vi "test_Packet_SimplePipelineResult.vi"(8 "error in (no error)":errorcluster) -> (0 "error out":errorcluster, 3 "Test Passed":bool)   [LabVIEW 2019]
uses:
  PhotonVisionLib/TypeDef/PhotonTrackedTargetType.ctl
  PhotonVisionLib/TypeDef/TargetCornerType.ctl
  <vilib>/Rock Robotics/WPI/ThirdParty/JAS_Junk/TrajLib/TRANSFORM2D.ctl
  <vilib>/Rock Robotics/WPI/ThirdParty/JAS_Junk/TrajLib/TRANSLATION2D.ctl
  <vilib>/Rock Robotics/WPI/ThirdParty/JAS_Junk/TrajLib/ROTATION2D.ctl
  PhotonVisionLib/PhotonVisionLib.lvlib
  <vilib>/Rock Robotics/WPI/ThirdParty/JAS_Junk/TrajLib/Trajectory_Library.lvlib
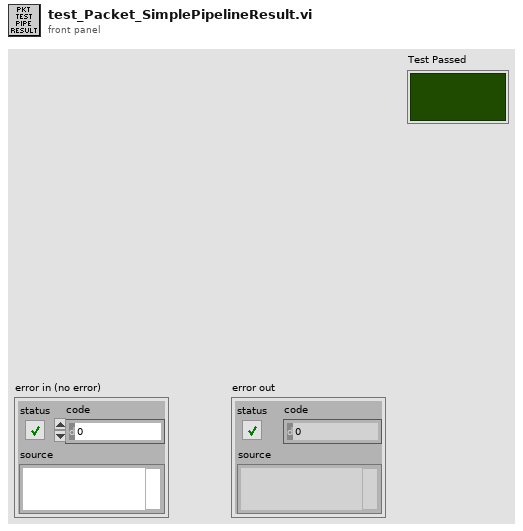
[diagram p1: front panel]
types:
  T1 = typedef "PhotonVisionLib.lvlib/PhotonTrackedTargetType.ctl" = cluster{"Yaw":dbl, "Pitch":dbl, "Area":dbl, "Skew":dbl, "TargetCorners":T2[], "CameraToTarget":T3}
  T2 = typedef "PhotonVisionLib.lvlib/TargetCornerType.ctl" = cluster{"X":dbl, "Y":dbl}
  T3 = typedef "Trajectory_Library.lvlib/TRANSFORM2D.ctl" = cluster{"TRANSLATION":T4, "ROTATION":T5}
  T4 = typedef "Trajectory_Library.lvlib/TRANSLATION2D.ctl" = cluster{"X":dbl, "Y":dbl}
  T5 = typedef "Trajectory_Library.lvlib/ROTATION2D.ctl" = cluster{"VALUE":dbl, "COS":dbl, "SIN":dbl}
  T6 = typedef "PhotonVisionLib.lvlib/PhotonPipelineResultType.ctl" = cluster{"TargetCount":i32, "Latency_MilliSec":dbl, "Targets":T1[]}
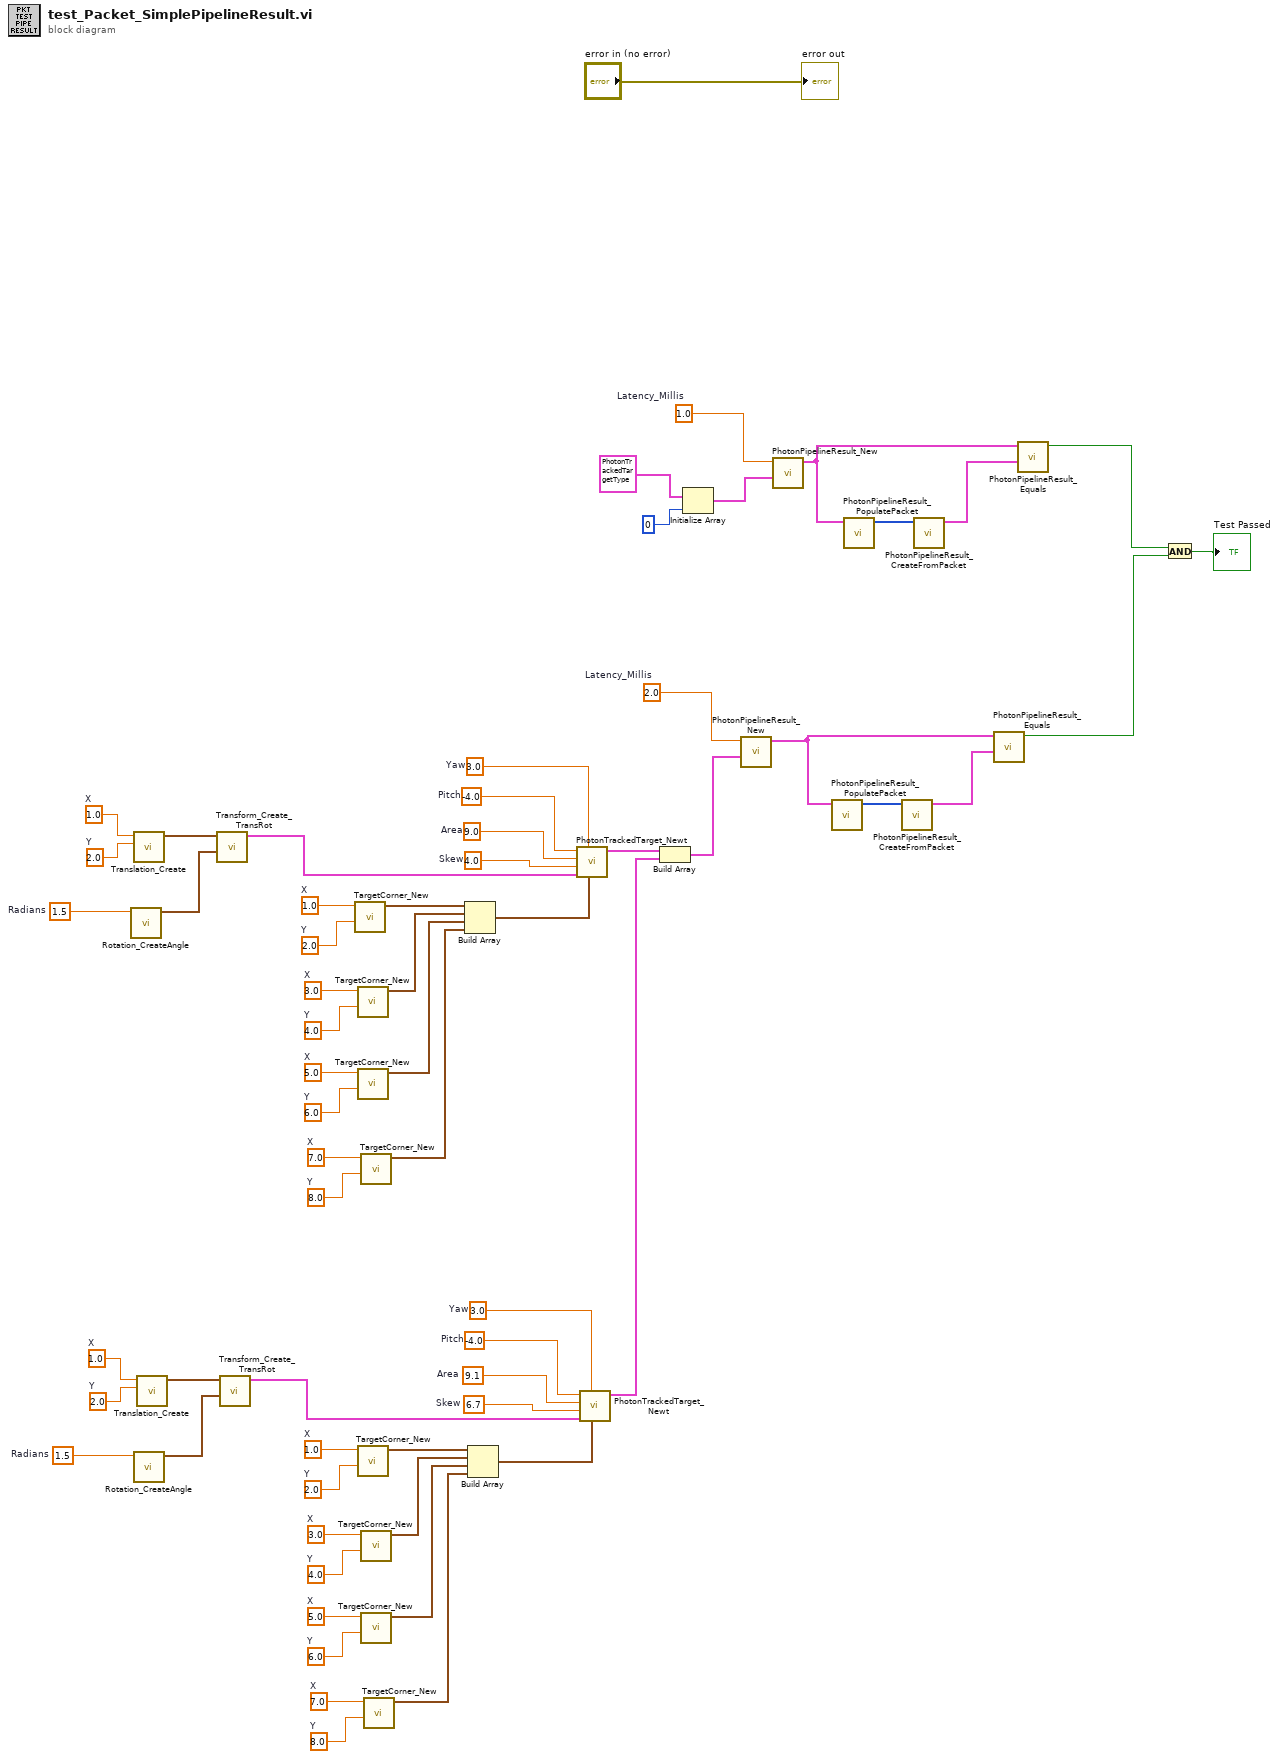
[diagram p0: block diagram]
diagram:
  w12 = 1.0  # Latency_Millis
  w14 = 2.0  # Latency_Millis
  w19 = 1.0  # X
  w20 = 2.0  # Y
  w22 = 1.5  # Radians
  w24 = -4.0  # Pitch
  w25 = 9.1  # Area
  w26 = 6.7  # Skew
  w27 = 3.0  # Yaw
  w33 = 7.0  # X
  w34 = 8.0  # Y
  w35 = 5.0  # X
  w36 = 6.0  # Y
  w37 = 3.0  # X
  w38 = 4.0  # Y
  w39 = 1.0  # X
  w40 = 2.0  # Y
  w42 = 1.0  # X
  w43 = 2.0  # Y
  w45 = 1.5  # Radians
  w47 = -4.0  # Pitch
  w48 = 9.0  # Area
  w49 = 4.0  # Skew
  w50 = 3.0  # Yaw
  w56 = 7.0  # X
  w57 = 8.0  # Y
  w58 = 5.0  # X
  w59 = 6.0  # Y
  w60 = 3.0  # X
  w61 = 4.0  # Y
  w62 = 1.0  # X
  w63 = 2.0  # Y
  n1 = call <vilib>:"Rotation_CreateAngle.vi"("Angle"=w45) -> ("ROTATION"=w44:T5)  [unwired: 10 in]
  n2 = call <vilib>:"Translation_Create.vi"("Y"=w43, "X"=w42) -> ("TRANSLATION"=w46:T4)  [unwired: 9 in]
  n3 = call <vilib>:"Rotation_CreateAngle.vi"("Angle"=w22) -> ("ROTATION"=w21:T5)  [unwired: 10 in]
  n4 = call <vilib>:"Translation_Create.vi"("Y"=w20, "X"=w19) -> ("TRANSLATION"=w23:T4)  [unwired: 9 in]
  n5 = call <vilib>:"Transform_Create_TransRot.vi"("ROTATION"=w44, "TRANSLATION"=w46) -> ("TRANSFORM"=w41:T3)  [unwired: 9 in]
  n6 = call <vilib>:"Transform_Create_TransRot.vi"("ROTATION"=w21, "TRANSLATION"=w23) -> ("TRANSFORM"=w18:T3)  [unwired: 9 in]
  n7 = call "TargetCorner_New.vi"("Y"=w63, "X"=w62) -> ("TargetCorner"=w55:T2)  [unwired: 9 in]
  n8 = call "TargetCorner_New.vi"("Y"=w61, "X"=w60) -> ("TargetCorner"=w53:T2)  [unwired: 9 in]
  n9 = call "TargetCorner_New.vi"("Y"=w59, "X"=w58) -> ("TargetCorner"=w52:T2)  [unwired: 9 in]
  n10 = call "TargetCorner_New.vi"("Y"=w40, "X"=w39) -> ("TargetCorner"=w32:T2)  [unwired: 9 in]
  n11 = call "TargetCorner_New.vi"("Y"=w57, "X"=w56) -> ("TargetCorner"=w51:T2)  [unwired: 9 in]
  n12 = call "TargetCorner_New.vi"("Y"=w38, "X"=w37) -> ("TargetCorner"=w30:T2)  [unwired: 9 in]
  n13 = call "TargetCorner_New.vi"("Y"=w36, "X"=w35) -> ("TargetCorner"=w29:T2)  [unwired: 9 in]
  n14 = call "TargetCorner_New.vi"("Y"=w34, "X"=w33) -> ("TargetCorner"=w28:T2)  [unwired: 9 in]
  n15 = Build Array(w55, w53, w52, w51) -> (w54:T2[])
  n16 = Build Array(w32, w30, w29, w28) -> (w31:T2[])
  n17 = call "PhotonTrackedTarget_Newt.vi"("TargetCorners"=w54, "Yaw"=w50, "CameraToTarget"=w41, "Skew"=w49, "Area"=w48, "Pitch"=w47) -> ("TrackedTarget"=w17:T1)  [unwired: 5 in]
  n18 = call "PhotonTrackedTarget_Newt.vi"("TargetCorners"=w31, "Yaw"=w27, "CameraToTarget"=w18, "Skew"=w26, "Area"=w25, "Pitch"=w24) -> ("TrackedTarget"=w16:T1)  [unwired: 5 in]
  n19 = Build Array(w17, w16) -> (w15:T1[])
  n20 = Initialize Array(T1 {"Yaw"=0.0, "Pitch"=0.0, "Area"=0.0, "Skew"=0.0, "TargetCorners"=[], "CameraToTarget"={"TRANSLATION"={"X"=0.0, "Y"=0.0}, "ROTATION"={"VALUE"=0.0, "COS"=1.0, "SIN"=0.0}}} ("PhotonTrackedTarget"), 0 ("dimension size")) -> (w9:T1[])
  n21 = call "PhotonPipelineResult_New.vi"("TrackedTargets"=w15, "Latency_Millis"=w14) -> ("PhotonPipelineResult"=w5:T6)  [unwired: 9 in]
  n22 = call "PhotonPipelineResult_New.vi"("TrackedTargets"=w9, "Latency_Millis"=w12) -> ("PhotonPipelineResult"=w7:T6)  [unwired: 9 in]
  n23 = call "PhotonPipelineResult_PopulatePacket.vi"("PhotonPipelineResult"=w5) -> ("Packet_RawData"=w13:u8[])  [unwired: 10 in]
  n24 = call "PhotonPipelineResult_PopulatePacket.vi"("PhotonPipelineResult"=w7) -> ("Packet_RawData"=w8:u8[])  [unwired: 10 in]
  n25 = call "PhotonPipelineResult_CreateFromPacket.vi"("RawData"=w13) -> ("PhotonPipelineResult"=w4:T6)  [unwired: 10 in]
  n26 = call "PhotonPipelineResult_CreateFromPacket.vi"("RawData"=w8) -> ("PhotonPipelineResult"=w6:T6)  [unwired: 10 in]
  n27 = call "PhotonPipelineResult_Equals.vi"("Other PhotonPipelineResult"=w4, "PhotonPipelineResult"=w5) -> ("Equal"=w1:bool)  [unwired: 9 in]
  n28 = call "PhotonPipelineResult_Equals.vi"("Other PhotonPipelineResult"=w6, "PhotonPipelineResult"=w7) -> ("Equal"=w2:bool)  [unwired: 9 in]
  n29 = And(x=w2, y=w1) -> (x .and. y?=→"Test Passed":bool)
  "error out" <- "error in (no error)"
